vi "DCA Calibration Verification.vi"(8 "error in (no error)":errorcluster, 9 "Calibration":T1) -> (0 "error out":errorcluster, 1 "Cal Accepted?":bool)   [LabVIEW 2011]
uses:
  TypeDefs/DCA Calibration State.ctl
panel:
  in  "B 1":bool
  in  "B 2":bool
  out "Cal Header":string="Normalization Offset = 0.000000"
  in  "Message (\"\")":string="The instrument normalization is complete.\n\nPlease select one of the following options:\n\n    Decline  -  start the calibration process over\n    Accept  -  accept the normalization offset and continue testing by\n                     following these steps:\n                     1)  Remove the short from the test fixtrue;\n                     2)  Place the part to be measured into the test fixture;\n                     3)  Press the Accept button to continue."
  # "(W)"
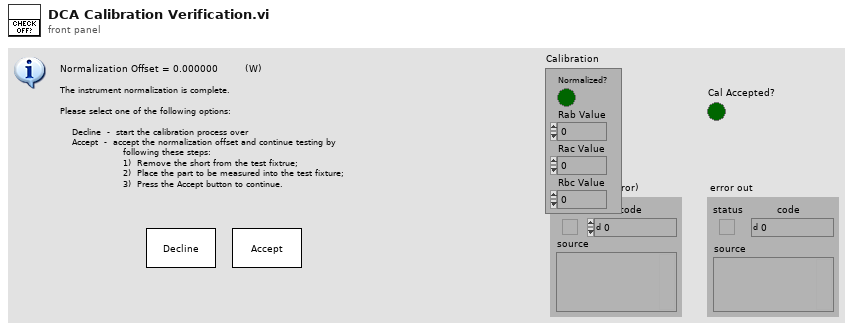
[diagram p1: front panel]
types:
  T1 = typedef "DCA Calibration State.ctl" = cluster{"Normalized?":bool, "Rab Value":dbl, "Rac Value":dbl, "Rbc Value":dbl}
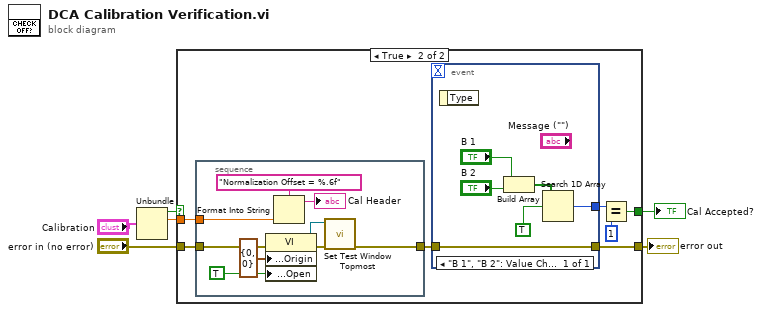
[diagram p0: block diagram]
diagram:
  n1 = Unbundle("Calibration") -> ("Normalized?"=w2:bool, "Rab Value"=w1:dbl)  [unwired: 2 out]
  n2 = case shown="True" w2 {
    selector: w2 -> [w8 _]
    tunnel: [w8 w10] -> w5
    tunnel: w1 -> [_ w14]
    tunnel: "error in (no error)" -> [w7 w13]
    tunnel: [w7 w9] -> w3
    frame False {
    }
    frame True {
      n3 = stacked-sequence {
        tunnel: w13 -> [w24]
        tunnel: [w21] -> w15
        tunnel: w14 -> [w17]
        frame #0 {
          n4 = property on="Property Node" class="VI"(error in=w24, "Front Panel Window:Origin"=cluster{"Horizontal":i16, "Vertical":i16} {"Horizontal"=0, "Vertical"=0}, "Front Panel Window:Open"=TRUE) -> (reference out=w20:refnum<vi>, error out=w22:errorcluster)  [unwired: 1 in]
          n5 = Format Into String(format string="Normalization Offset = %.6f", w17) -> (resulting string=→"Cal Header":string)  [unwired: 2 in, 1 out]
          n6 = call "Set Test Window Topmost.vi"("error in (no error)"=w22, "VI Refnum"=w20) -> ("error out"=w21:errorcluster)  [unwired: 5 out]
        }
      }
      n7 = event shown="[0] \"B 1\", \"B 2\": Value Change" {
        selector: _ -> [_]
        dyn-events: _ -> [_]
        timeout: _ -> [_]
        tunnel: w15 -> [w30]
        tunnel: [w30] -> w9
        tunnel: [w25] -> w12
        event "B 1", "B 2": Value Change {
          n8 = event-data() -> ()  [unwired: 2 out]
          n9 = Build Array("B 1", "B 2") -> (w27:bool[])
          n10 = Search 1D Array(1D array=w27, element=TRUE) -> (index of element=w25:i32)  [unwired: 1 out]
        }
      }
      n11 = Equal?(x=w12, y=1) -> (x = y?=w10:bool)
    }
  }
  "error out" <- w3
  "Cal Accepted?" <- w5
